vi "CC RA and DEC to decimal.vi"(8 "error in (no error)":errorcluster, 11 "RA and DEC String":cluster{"RA":string, "DEC":string}={"RA"="HH:MM:SS.nnn", "DEC"="DEG:arcmin:arcsec.nn"} caption="RA and DEC") -> (0 "error out":errorcluster, 3 "RA and DEC":T1)   [LabVIEW 2024]
uses:
  typedefs/CC cluster RA and DEC.ctl
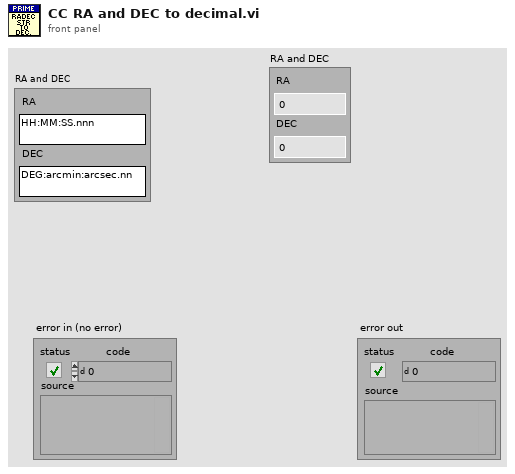
[diagram p1: front panel]
types:
  T1 = typedef "CC cluster RA and DEC.ctl" = cluster{"RA":dbl, "DEC":dbl}
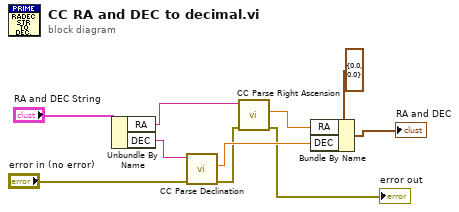
[diagram p0: block diagram]
diagram:
  n1 = Unbundle By Name("RA and DEC String") -> ("RA"=w9:string, "DEC"=w8:string)
  n2 = call "CC Parse Declination.vi"("error in (no error)"="error in (no error)", "Declination string"=w8) -> ("error out"=w2:errorcluster, "Angle"=w5:dbl)  [unwired: 7 in, 1 out]
  n3 = call "CC Parse Right Ascension.vi"("error in (no error)"=w2, "Right Ascension string"=w9) -> ("error out"=→"error out":errorcluster, "Angle"=w6:dbl)  [unwired: 7 in, 1 out]
  n4 = Bundle By Name(cluster=T1 {"RA"=0.0, "DEC"=0.0} ("RA and DEC"), "RA"=w6, "DEC"=w5) -> (→"RA and DEC":T1)
